vi "HelperLabelText.vi"(0 "Text in":refnum<vi>) -> (1 "Text":string)   [LabVIEW 2013]
panel:
  out "error out":errorcluster
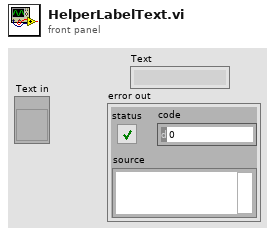
[diagram p1: front panel]
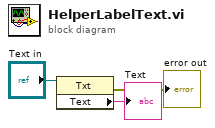
[diagram p0: block diagram]
diagram:
  n1 = property class="Txt"(reference="Text in") -> (error out=→"error out":errorcluster, "Text"=→"Text":string)  [unwired: 1 in, 1 out]
